vi "Sum array.vi"(1 "Array in":dbl[](array[numeric])) -> (0 "Sum":dbl)   [LabVIEW 2015]
panel:
  out "Test Point 3":dbl[](array[numeric])
  out "Test Point 2":dbl[](array[numeric])
  out "Test Point 1":dbl[](array[numeric])
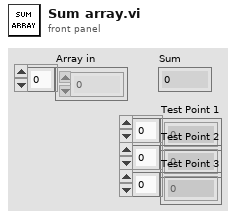
[diagram p1: front panel]
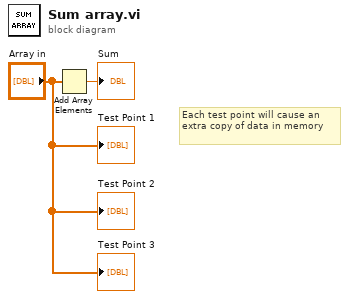
[diagram p0: block diagram]
diagram:
  # "Each test point will cause an extra copy of data in memory"
  n1 = Add Array Elements(numeric array="Array in") -> (sum=→"Sum":dbl)
  "Test Point 1" <- "Array in"
  "Test Point 2" <- "Array in"
  "Test Point 3" <- "Array in"
